vi "CAN1_2AccVal.vi"() -> ()   [LabVIEW 2011]
doc: "This example demonstrates receiving frames using an NI-XNET Frame Input session. \n\nThis examples is made to be run against the CAN Frame Output Single Point example, assuming you have a properly terminated CAN cable connected to two CAN ports.\n\nIf you do not have any database aliases on your system, the example will automatically load the nixnet_example database."
uses:
  <vilib>/Platform/TimedLoop/XDataNode/timing_clust.ctl
  <vilib>/Platform/TimedLoop/XDataNode/nitl_modes.ctl
  <vilib>/Platform/TimedLoop/XDataNode/wakeup.ctl
  <vilib>/xnet/xnet.llb/XNET Read (Frame CAN).vi
  <vilib>/Platform/TimedLoop/XDataNode/XDataNode.xnode
  <vilib>/Platform/TimedLoop/XDataNode/XDNodeRunTimeDep.lvlib
panel:
  out "element":i16
  in  "Numeric":dbl
  out "Waveform Chart 3":i16(graph)
  out "Waveform Chart 2":cluster{i16, i16, i16}(graph)
  in  "stop":bool
  # "For instructions, select Help>>Show Context Help and drag your mouse over the VI icon on the top right."
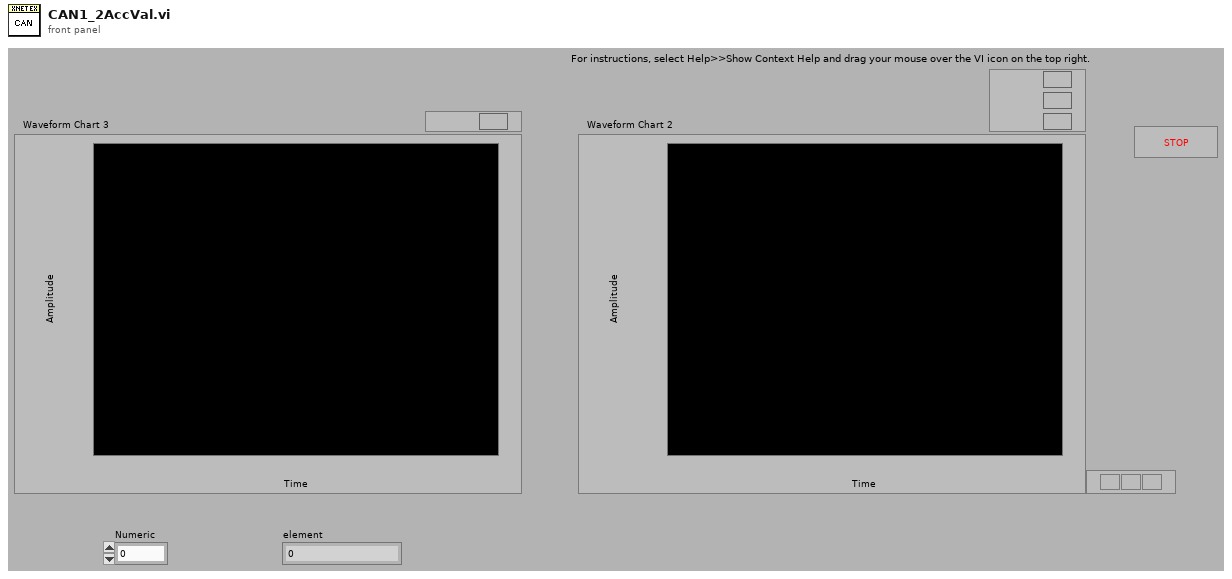
[diagram p1: front panel]
types:
  T1 = typedef "XDNodeRunTimeDep.lvlib/timing_clust.ctl" = cluster{"Expected End [f-1]":u64, "Actual End [f-1]":u64, "Finished Late? [f-1]":bool, "Expected End [i-1]":u64, "Actual End [i-1]":u64, "Finished Late? [i-1]":bool, "Expected Start [i]":u64, "Actual Start [i]":u64, "Expected Start [f]":u64, "Actual Start [f]":u64, "Source Name":string, "Structure Name":string, "Period":i64, "Deadline":i64, "Offset":i64, "Start":i64, "Priority":i32, "Timeout":i32, "Mode":T2, "Wakeup Reason":T3, "Error":errorcluster, "Source Type":string, "Secondary Source Type":string, "Global End Time":u64, "Global Start Time":u64, "Frame Duration":u64, "Iteration Duration":u64, "Assigned CPU":i32, "I/O Scan Engine Mode":u32}
  T2 = typedef "XDNodeRunTimeDep.lvlib/nitl_modes.ctl" = enum32{"No Change", "Process missed periods, maintain original phase", "Discard missed periods, maintain original phase", "Process missed periods, ignore original phase", "Discard missed periods, ignore original phase"}
  T3 = typedef "XDNodeRunTimeDep.lvlib/wakeup.ctl" = enum32{"Normal", "Aborted", "Asynchronous wakeup", "Timing source error", "Timed loop error", "Timeout"}
  T4 = typedef "XNET Frame CAN.ctl" = cluster{"timestamp":timestamp, "payload":u8[], "identifier":u32, "type":T5, "extended?":bool, "echo?":bool}
  T5 = typedef "XNET Frame Type CAN.ctl" = u8
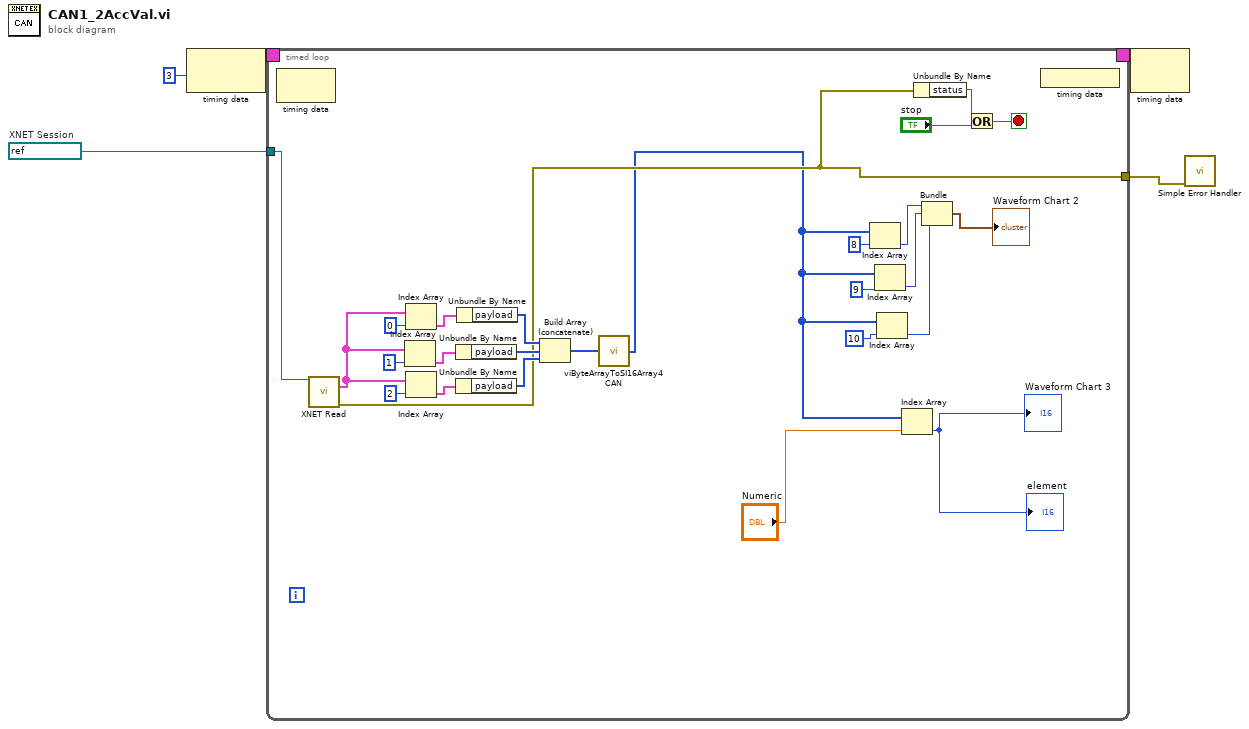
[diagram p0: block diagram]
diagram:
  w1 = refnum<k21> "iTremCan"  # XNET Session
  n1 = node-c288(i64 3 ("Period")) -> (w5:T1)
  n2 = timed-loop {
    tunnel: w1 -> [w10]
    tunnel: [w9] -> w3
    timing: w5 -> [_]
    timing-out: [_] -> w4
    stop <- w29 stop-if-true
    n3 = node-c288() -> ()  [unwired: 2 out]
    n4 = call-poly <vilib>:"XNET Read.vi"("session in"=w10) -> ("data"=w17:T4[], "error out"=w9:errorcluster)  [unwired: 1 in, 12 out]
    n5 = Index Array(array=w17, index=1) -> (element=w15:T4)
    n6 = Index Array(array=w17, index=0) -> (element=w16:T4)
    n7 = Index Array(array=w17, index=2) -> (element=w14:T4)
    n8 = Unbundle By Name(w15) -> ("payload"=w12:u8[])
    n9 = Unbundle By Name(w14) -> ("payload"=w11:u8[])
    n10 = Unbundle By Name(w16) -> ("payload"=w13:u8[])
    n11 = Build Array (concatenate)(w13, w12, w11) -> (w8:u8[])
    n12 = call "viByteArrayToSI16Array4CAN.vi"("input variable"=w8) -> ("output variable"=w7:i16[])
    n13 = Index Array(array=w7, index=8) -> (element=w27:i16)
    n14 = Index Array(array=w7, index=9) -> (element=w24:i16)
    n15 = Index Array(array=w7, index=10) -> (element=w23:i16)
    n16 = Index Array(array=w7, index="Numeric") -> (element=→"Waveform Chart 3" →"element":i16)
    n17 = Unbundle By Name(w9) -> ("status"=w31:bool)
    n18 = Bundle(w27, w24, w23) -> (→"Waveform Chart 2":cluster{i16, i16, i16})  [unwired: 1 in]
    n19 = Or(x=w31, y="stop") -> (x .or. y?=w29:bool)
    n20 = node-c288() -> ()  [unwired: 1 out]
  }
  n21 = node-c288(w4) -> ()  [unwired: 1 out]
  n22 = call <vilib>:"Simple Error Handler.vi"("error in (no error)"=w3) -> ()  [unwired: 1 in, 8 out]
